vi "Release Host Key.vi"(8 "error in (no error)":errorcluster, 11 "host key":T1) -> (0 "error out":errorcluster)   [LabVIEW 2017, in "libssh2.lvlib"]
doc: "Release the memory associated with a host key."
uses:
  libssh2.lvlib
  Host Key Refnum.ctl
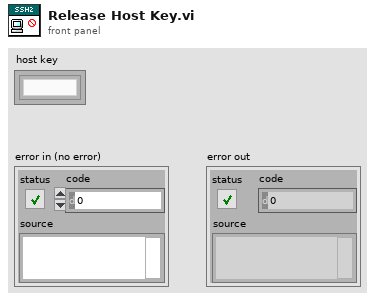
[diagram p1: front panel]
types:
  T1 = typedef "libssh2.lvlib/Host Key Refnum.ctl" = refnum<k1>
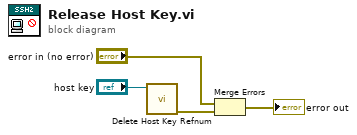
[diagram p0: block diagram]
diagram:
  n1 = call "Delete Host Key Refnum.vi"("host key"="host key") -> ("error out"=w3:errorcluster)  [unwired: 9 in, 1 out]
  n2 = Merge Errors("error in (no error)", w3) -> (→"error out":errorcluster)
